vi "CD Engine lvlib.vi"(8 "error in (no error)":errorcluster, 9 "Action":T1) -> (0 "error out":errorcluster, 1 "Output":string)   [LabVIEW 2014, in "CD model script.lvlib"]
doc: "Constants, which are necessary for the <B>CD Engine library</B> in the generated custom device project."
uses:
  CD model script.lvlib
  Constants TypDef/CD Engine lvlib.ctl
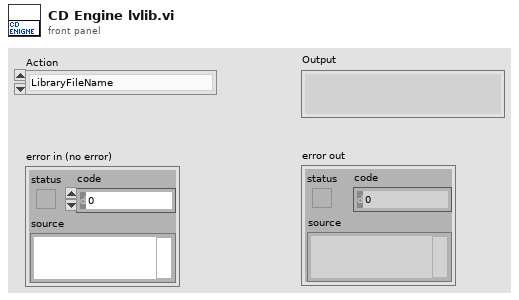
[diagram p1: front panel]
types:
  T1 = typedef "CD model script.lvlib/CD Engine lvlib.ctl" = enum16{"LibraryFileName", "LibraryFolderName", "Engine.FolderName", "Engine.Init.FolderName", "Engine.Run.FolderName", "Engine.Shutdown.FolderName", "Types.FolderName", "Engine.RT Driver VI.TemplatePath", "Engine.RT Driver VI.FileName"}
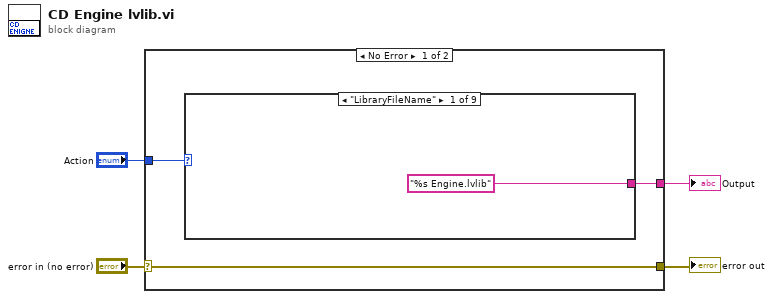
[diagram p0: block diagram]
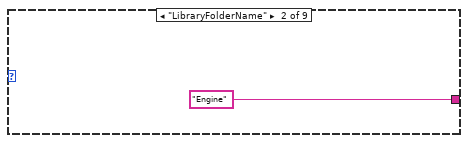
[diagram p2: hidden frame]
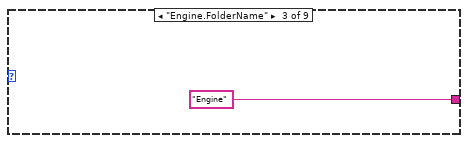
[diagram p3: hidden frame]
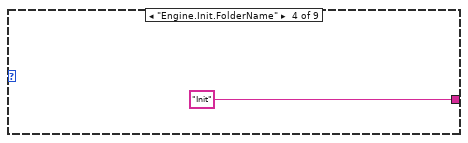
[diagram p4: hidden frame]
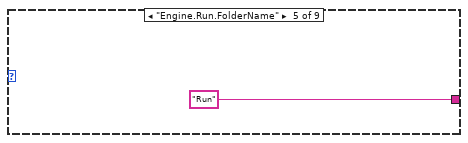
[diagram p5: hidden frame]
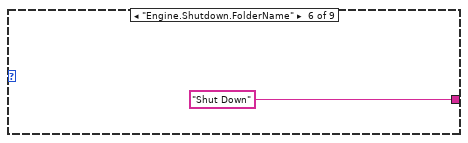
[diagram p6: hidden frame]
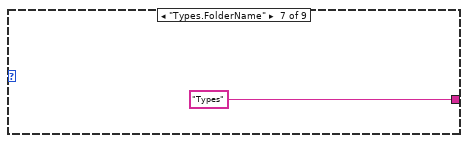
[diagram p7: hidden frame]
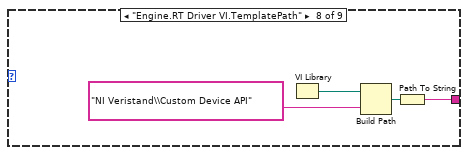
[diagram p8: hidden frame]
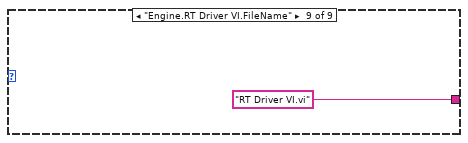
[diagram p9: hidden frame]
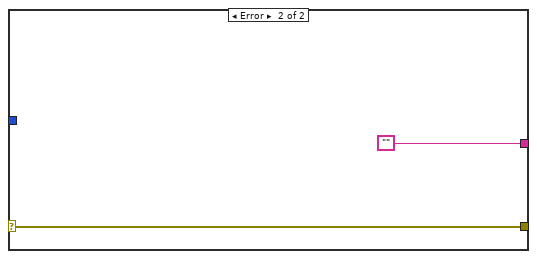
[diagram p10: hidden frame]
diagram:
  n1 = case shown="No Error" "error in (no error)" {
    selector: "error in (no error)" -> [w7 w21]
    tunnel: [w7 w21] -> w1
    tunnel: [w5 ""] -> w2
    tunnel: "Action" -> [w6 _]
    frame No Error {
      n2 = case shown="\"LibraryFileName\"" w6 {
        tunnel: ["%s Engine.lvlib" "Engine" "Engine" "Init" "Run" "Shut Down" "Types" w15 "RT Driver VI.vi"] -> w5
        frame "LibraryFileName" {
        }
        frame "LibraryFolderName" {
        }
        frame "Engine.FolderName" {
        }
        frame "Engine.Init.FolderName" {
        }
        frame "Engine.Run.FolderName" {
        }
        frame "Engine.Shutdown.FolderName" {
        }
        frame "Types.FolderName" {
        }
        frame "Engine.RT Driver VI.TemplatePath" {
          n3 = VI Library() -> (path=w16:path)
          n4 = Build Path(base path=w16, name or relative path="NI Veristand\\Custom Device API") -> (appended path=w18:path)
          n5 = Path To String(path=w18) -> (string=w15:string)
        }
        frame "Engine.RT Driver VI.FileName" {
        }
      }
    }
    frame Error {
    }
  }
  "error out" <- w1
  "Output" <- w2
